vi "Add Message.vi"(0 "PainOutputTerminal in":refnum<class "PainOutputTerminal.lvclass">, 5 "Line Number":i64, 7 "Message":string, 11 "error in (no error)":errorcluster) -> (4 "PainOutputTerminal out":refnum<class "PainOutputTerminal.lvclass">, 15 "error out":errorcluster)   [LabVIEW 2019, in "PainOutputTerminal.lvclass"]
uses:
  PainOutputTerminal.lvclass
  PainOutputTerminal.lvclass/PainOutputTerminal.ctl
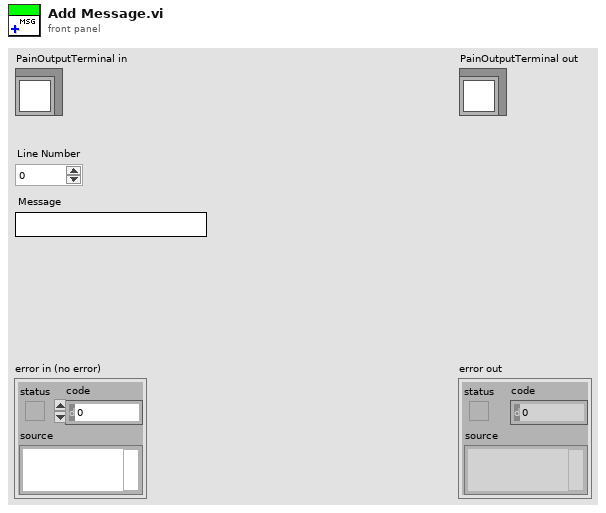
[diagram p1: front panel]
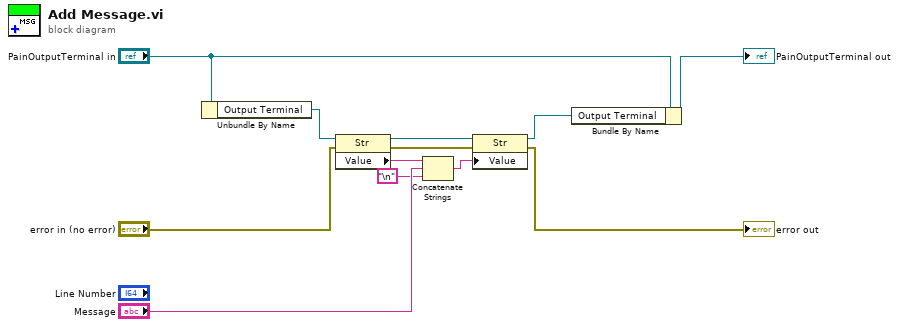
[diagram p0: block diagram]
diagram:
  n1 = Unbundle By Name("PainOutputTerminal in") -> ("Output Terminal"=w11:refnum<vi>)
  n2 = property class="Str"(reference=w11, error in="error in (no error)") -> (reference out=w10:refnum<vi>, error out=w12:errorcluster, "Value"=w8:string)
  n3 = Concatenate Strings(w8, "Message", "\n" ("string")) -> (w7:string)
  n4 = property class="Str"(reference=w10, error in=w12, "Value"=w7) -> (reference out=w9:refnum<vi>, error out=→"error out":errorcluster)
  n5 = Bundle By Name(cluster="PainOutputTerminal in", "Output Terminal"=w9) -> (→"PainOutputTerminal out":refnum<class "PainOutputTerminal.lvclass">)
